vi "Subtractor2.vi"() -> (8 "Subtractor2":refnum<class "Subtractor2.lvclass">)   [LabVIEW 2017, in "Subtractor2.lvclass"]
uses:
  Subtractor2.lvclass
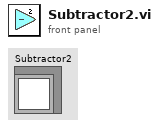
[diagram p1: front panel]
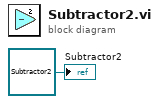
[diagram p0: block diagram]
diagram:
  "Subtractor2" <- refnum<class "Subtractor2.lvclass"> refnum ("Subtractor2.lvclass")
